vi "Launch Async Auth.vi"(5 "Refresh Only?":bool, 6 "Failed HTML Response":string="<html><body><h1>Failed</h1><p>Please close this page and return to the application</p></body></html>", 7 "Success HTML Response":string="<html><body><h1>Success</h1><p>You can close this page and return to the application.</p></body></html>", 8 "error in (no error)":errorcluster, 9 "Timeout S (60)":dbl=60.0, 10 "Authorization in":refnum<class "Authorization.lvclass">, 11 "OAuth2 in":refnum<class "OAuth2.lvclass">) -> (0 "error out":errorcluster, 1 "Async Authentication":refnum<class "Async Authorization.lvclass">, 3 "OAuth2 out":refnum<class "OAuth2.lvclass">)   [LabVIEW 2020, in "OAuth2.lvlib" / "OAuth2.lvclass"]
uses:
  OAuth2.lvclass
  OAuth2.lvclass/OAuth2.ctl
  Auth Async.vi
  Async Authorization/Async Authorization.lvclass
  HTTP Utils/Response/Response.lvclass
  Authorization/Authorization.lvclass
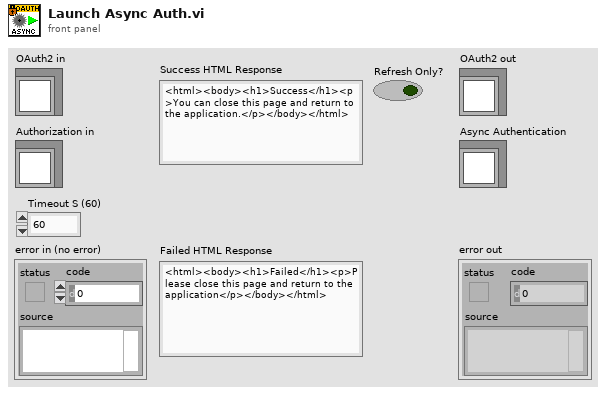
[diagram p1: front panel]
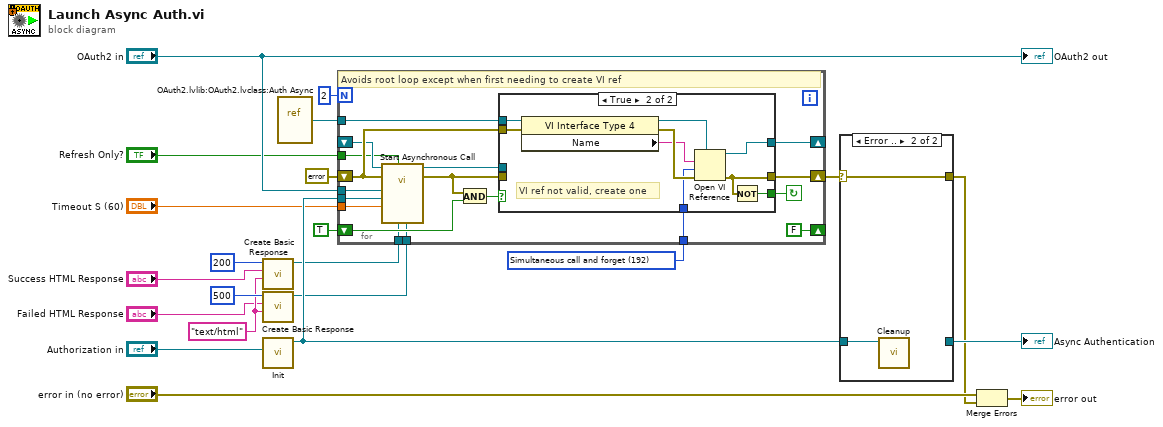
[diagram p0: block diagram]
diagram:
  w6 = "text/html" ("Content-Type (text/plain)")
  w19 = 192 items=["Record modifications"=1, "Open templates for editing"=2, "Prompt user to save"=4, "Prepare for reentrant run"=8, "Prompt to find missing subVIs"=16, "Hide loading dialog box"=32, "Enable simultaneous calls"=64, "Prepare to call and forget"=128, "Simultaneous call and forget"=192, "Prepare to call and collect"=256, "Simultaneous call and collect"=320]
  n1 = call "Create Basic Response.vi"("Content-Type (text/plain)"=w6, "Payload"="Success HTML Response", "Status Code"=u16 200) -> ("Response out"=w3:refnum<class "Response.lvclass">)  [unwired: 7 in, 1 out]
  n2 = call "Create Basic Response.vi"("Content-Type (text/plain)"=w6, "Payload"="Failed HTML Response", "Status Code"=u16 500) -> ("Response out"=w2:refnum<class "Response.lvclass">)  [unwired: 7 in, 1 out]
  n3 = call "Init.vi"("Authorization"="Authorization in") -> ("Async Authorization out"=w13:refnum<class "Async Authorization.lvclass">)  [unwired: 9 in, 1 out]
  n4 = vi-ref "OAuth2.lvlib:OAuth2.lvclass:Auth Async.vi"() -> (w18:refnum<vi>)
  n5 = for {
    N: 2 -> [_]
    tunnel: w18 -> [w39]
    tunnel: w19 -> [w38]
    shift-right: [w37] -> _
    shift-left: _ -> [w36]
    shift-right: [w34] -> w14
    shift-left: errorcluster {"status"=FALSE, "code"=0, "source"=""} ("error constant") -> [w40]
    shift-right: [FALSE] -> _
    shift-left: TRUE -> [w31]
    tunnel: "OAuth2 in" -> [w28]
    tunnel: w13 -> [w27]
    tunnel: "Timeout S (60)" -> [w26]
    tunnel: w3 -> [w25]
    tunnel: w2 -> [w24]
    tunnel: "Refresh Only?" -> [w23]
    stop <- w30 continue-if-true
    # "Avoids root loop except when first needing to create VI ref"
    n6 = call-by-ref "Start Asynchronous Call"(reference=w36, error in=w40, "Failed Response"=w24, "Complete Response"=w25, "Refresh Only?"=w23, "Timeout S"=w26, "Async Authorization"=w27, "OAuth2 in"=w28) -> (reference out=w35:refnum<vi>, error out=w33:errorcluster)  [unwired: 6 in]
    n7 = And(x=w33, y=w31) -> (x .and. y?=w32:bool)
    n8 = case shown="True" w32 {
      tunnel: w39 -> [_ w50]
      tunnel: w38 -> [_ w48]
      tunnel: [w42 w46] -> w37
      tunnel: w35 -> [w42 _]
      tunnel: [w41 w44] -> w34
      tunnel: w33 -> [w41 _]
      tunnel: w40 -> [_ w45]
      tunnel: [_ w43] -> w30
      frame False {
        # "Keep reusing valid VI ref"
      }
      frame True {
        # "VI ref not valid, create one"
        n9 = property class="VI Interface Type 4"(reference=w50, error in=w45) -> (reference out=w47:refnum<vi>, error out=w51:errorcluster, "Name"=w49:string)
        n10 = Open VI Reference(type specifier VI Refnum (for type only)=w47, vi path=w49, options=w48, error in (no error)=w51) -> (vi reference=w46:refnum<vi>, error out=w44:errorcluster)  [unwired: 2 in]
        n11 = Not(x=w44) -> (.not. x?=w43:bool)
      }
    }
  }
  n12 = case shown="Error .." w14 {
    selector: w14 -> [_ w53]
    tunnel: w13 -> [w52 w54]
    tunnel: [w52 _] -> w12
    tunnel: [_ w53] -> w10
    frame No Error {
    }
    frame Error {
      n13 = call "Cleanup.vi"("Async Authorization in"=w54) -> ()  [unwired: 10 in, 1 out]
    }
  }
  "Async Authentication" <- w12
  n14 = Merge Errors("error in (no error)", w10) -> (→"error out":errorcluster)
  "OAuth2 out" <- "OAuth2 in"
